vi "Laurel Meter TCP.vi"(0 "TCP Network Connection in":refnum<k5>, 1 "Laurel Serial Commands":T3, 2 "Serial VISA":refnum<visa-resource-name>, 5 "Connection Type":T2, 11 "error in (no error)":errorcluster, 12 "byte count (Individual)":i32=9, 13 "Display Type":T1, 14 "All Items Byte Count (Flow Rate)":i32=17) -> (3 "read buffer":string, 4 "TCP Network Connection out":refnum<k5>, 6 "Flow Rate (Item 1)":dbl format="%.2f", 8 "Serial VISA Out":refnum<visa-resource-name>, 9 "Single Item":dbl, 10 "Gallons (Item 2)":dbl, 15 "error out":errorcluster)   [LabVIEW 2020]
doc: "This VI uses a TCP Connection to the Laurel Meter. The port is the Standard Modbus 502 port"
uses:
  Type Definitions/Laurel Serial Commands.ctl
  Type Definitions/Laurel Connection Type.ctl
  Type Definitions/Laurel Display Type.ctl
panel:
  out "return count":i32
  # "Laurel Meter Setup"
  # "Ethernet"
  # "Power Input"
  # "Item 2"
  # "Manual\nReset"
  # "Item 1"
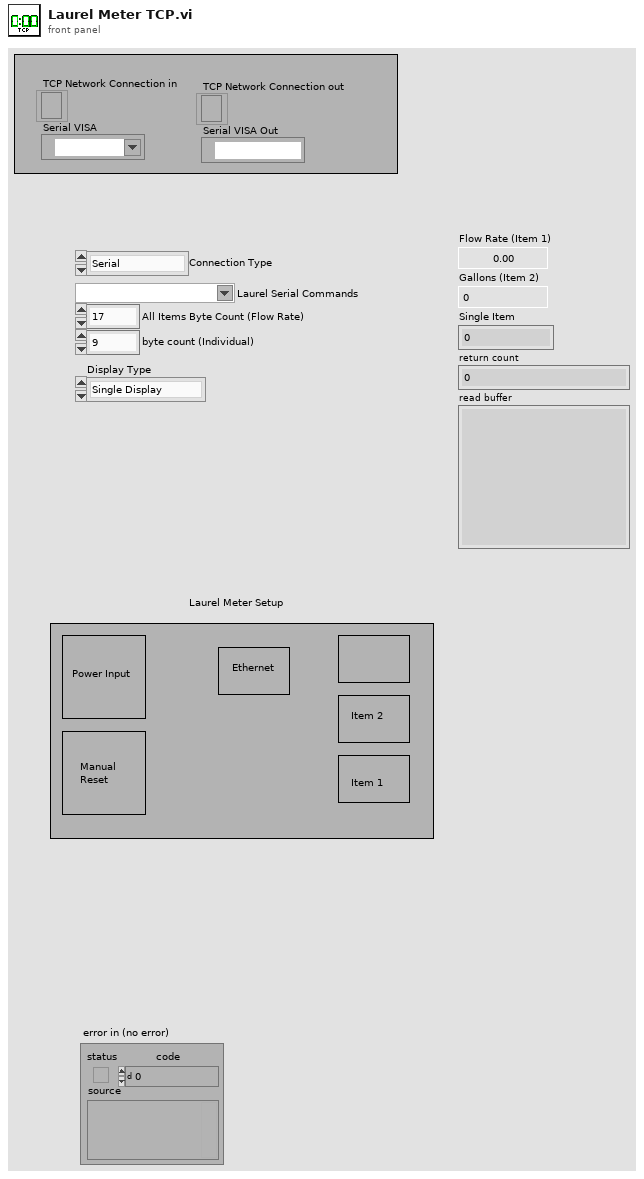
[diagram p1: front panel]
types:
  T1 = typedef "Laurel Display Type.ctl" = enum16{"Single Display", "Dual Display"}
  T2 = typedef "Laurel Connection Type.ctl" = enum16{"Serial", "TCP"}
  T3 = typedef "Laurel Serial Commands.ctl" = string
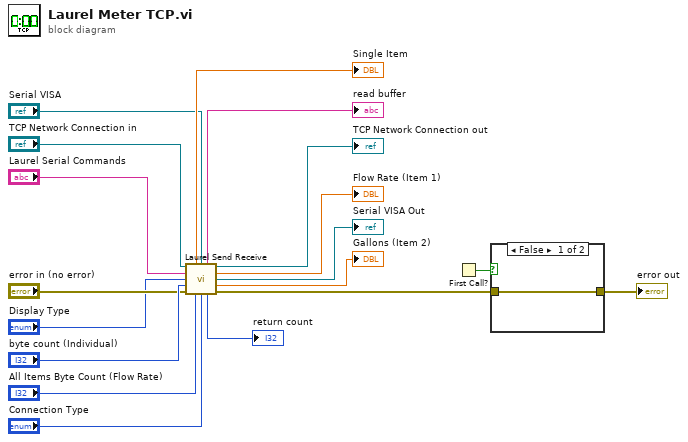
[diagram p0: block diagram]
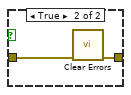
[diagram p2: hidden frame]
diagram:
  n1 = call "Laurel Send Receive.vi"("TCP Network Connection in"="TCP Network Connection in", "Serial VISA (Input)"="Serial VISA", "Laurel Serial Commands"="Laurel Serial Commands", "Display Type"="Display Type", "Individual Byte Count"="byte count (Individual)", "error in (no error)"="error in (no error)", "All Items Byte Count (Flow Rate)"="All Items Byte Count (Flow Rate)", "Connection Type"="Connection Type") -> ("Single Item"=→"Single Item":dbl, "Output String"=→"read buffer":string, "TCP Network Connection out"=→"TCP Network Connection out":refnum<k5>, "Flow Rate (Item 1)"=→"Flow Rate (Item 1)":dbl, "Serial VISA (Output)"=→"Serial VISA Out":refnum<visa-resource-name>, "Gallons (Item 2)"=→"Gallons (Item 2)":dbl, "return count"=→"return count":i32, "error out"=w9:errorcluster)
  n2 = First Call?() -> (First Call?: T/F=w10:bool)
  n3 = case shown="False" w10 {
    tunnel: w9 -> [w19 w21]
    tunnel: [w19 w20] -> w8
    frame False {
    }
    frame True {
      n4 = call <vilib>:"Clear Errors.vi"("error in (no error)"=w21) -> ("error out"=w20:errorcluster)  [unwired: 5 in, 1 out]
    }
  }
  "error out" <- w8
